vi "SetShiftSpeed.vi"() -> ()   [LabVIEW 2016]
uses:
  <userlib>/atmcd64d.llb/HSSpeed_type typedef.ctl
panel:
  in  "Set VSS":i32
  out "Allowed \nVertical \nShift Speed\n(MHz)":sgl[](array[numeric])
  in  "stop":bool
  in  "Set HSS":i32
  out "Allowed \nHorizontal \nShift Speed\n(MHz)":sgl[](array[numeric])
  out "model":string
  out "DLL error code from ini":u32
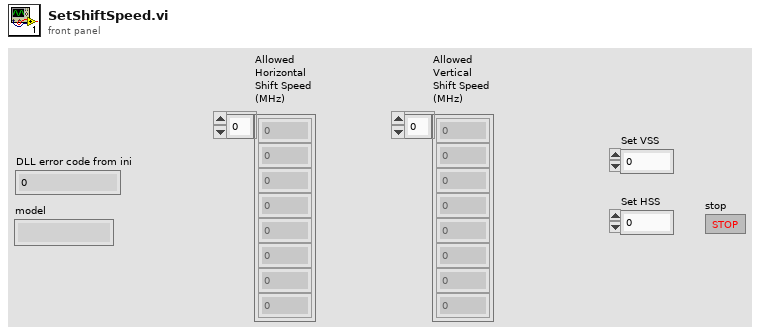
[diagram p1: front panel]
types:
  T1 = typedef "HSSpeed_type typedef.ctl" = enum16{"EM Amp", "Conventional Amp"}
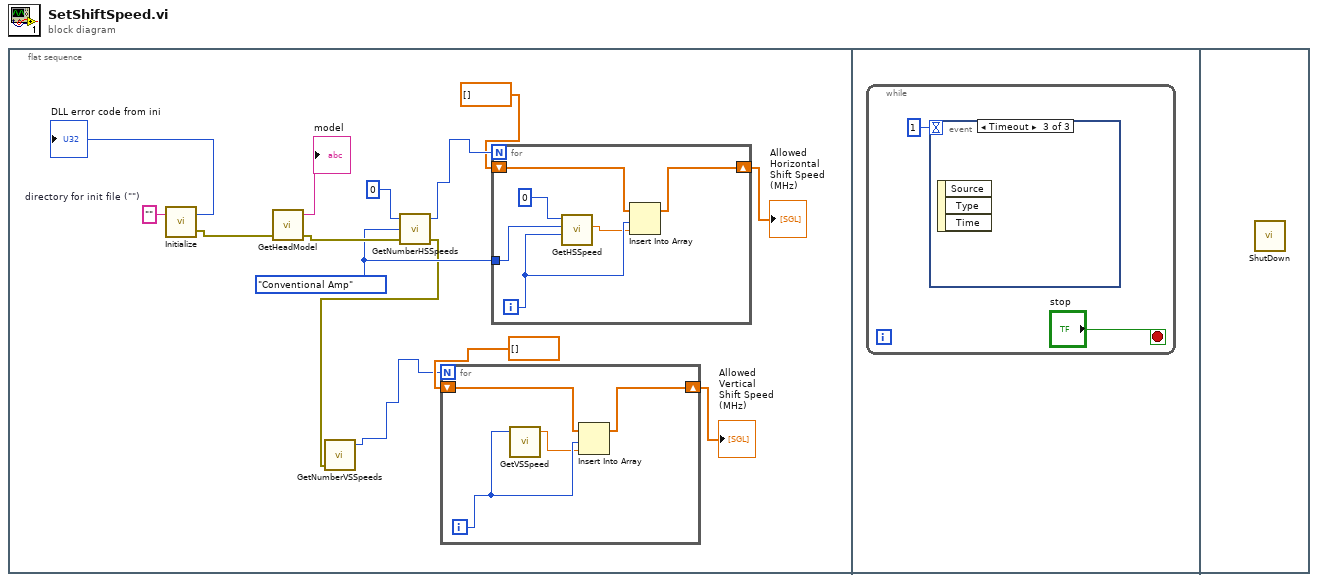
[diagram p0: block diagram]
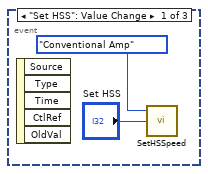
[diagram p2: hidden frame]
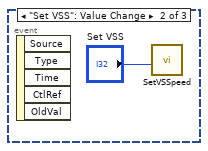
[diagram p3: hidden frame]
diagram:
  n1 = flat-sequence {
    frame #0 {
      w8 = HSSpeed_type_typedef."Conventional Amp" ("type")
      w14 = ""  # directory for init file ("")
      n2 = call <userlib>:"Initialize.vi"("directory (\"\")"=w14) -> ("error out"=w11:errorcluster, "DLL error code"=→"DLL error code from ini":u32)  [unwired: 1 in]
      n3 = call <userlib>:"GetHeadModel.vi"("error in (no error)"=w11) -> ("error out"=w10:errorcluster, "model"=→"model":string)  [unwired: 2 in, 1 out]
      n4 = call <userlib>:"GetNumberHSSpeeds.vi"("error in (no error)"=w10, "type"=w8, "channel"=0) -> ("error out"=w1:errorcluster, "number"=w7:i32)  [unwired: 1 out]
      n5 = call <userlib>:"GetNumberVSSpeeds.vi"("error in (no error)"=w1) -> ("number"=w2:i32)  [unwired: 2 in, 2 out]
      n6 = for {
        N: w2 -> [_]
        shift-right: [w17] -> w3
        shift-left: sgl[] [] -> [w18]
        i -> [w16]
        n7 = call <userlib>:"GetVSSpeed.vi"("index"=w16) -> ("speed"=w15:sgl)  [unwired: 2 in, 2 out]
        n8 = Insert Into Array(array=w18, index=w16, new element=w15) -> (w17:sgl[])
      }
      "Allowed \nVertical \nShift Speed\n(MHz)" <- w3
      n9 = for {
        N: w7 -> [_]
        tunnel: w8 -> [w21]
        shift-right: [w19] -> w5
        shift-left: sgl[] [] -> [w20]
        i -> [w24]
        n10 = call <userlib>:"GetHSSpeed.vi"("index"=w24, "type"=w21, "channel"=0) -> ("speed"=w23:sgl)  [unwired: 2 in, 2 out]
        n11 = Insert Into Array(array=w20, index=w24, new element=w23) -> (w19:sgl[])
      }
      "Allowed \nHorizontal \nShift Speed\n(MHz)" <- w5
    }
    frame #1 {
      n12 = while {
        stop <- "stop" stop-if-true
        n13 = event shown="[2] Timeout" {
          selector: _ -> [_ _ _]
          dyn-events: _ -> [_ _ _]
          timeout: 1 -> [_ _ _]
          event "Set HSS": Value Change {
            n14 = event-data() -> ()  [unwired: 1 in, 5 out]
            n15 = call <userlib>:"SetHSSpeed.vi"("index"="Set HSS", "type"=HSSpeed_type_typedef."Conventional Amp") -> ()  [unwired: 2 in, 2 out]
          }
          event "Set VSS": Value Change {
            n16 = event-data() -> ()  [unwired: 1 in, 5 out]
            n17 = call <userlib>:"SetVSSpeed.vi"("index"="Set VSS") -> ()  [unwired: 1 in, 2 out]
          }
          event Timeout {
            n18 = event-data() -> ()  [unwired: 1 in, 3 out]
          }
        }
      }
    }
    frame #2 {
      n19 = call <userlib>:"ShutDown.vi"() -> ()  [unwired: 2 in, 2 out]
    }
  }
